vi "Stop Core.vi"(10 "final error code":i32, 11 "DataBase in":refnum<class "DataBase.lvclass">) -> (3 "DataBase out":refnum<class "DataBase.lvclass">)   [LabVIEW 2019, in "DataBase.lvlib" / "DataBase.lvclass"]
doc: "(<B>Filename</B>: Actor Framework.lvlib:Actor.lvclass:Stop Core.vi)\n\nDefines what the actor does before it stops. Use the <B>final error code</B> input to determine whether the actor shut down in response to an error.\n\nBy default, this method passes the Stop message along to all auto-stop nested actors. A descendant class may override this method to define additional behavior, such as shutting down any processes the actor initiated in its override of the Actor Core method."
uses:
  DataBase.lvclass
  DataBase.lvclass/DataBase.ctl
  79d7bb73-9b32-4418-8980-8c007c1ce44f.vi
  <vilib>/NI/Event Source Actor/Event Source/Event Source/Event Source.lvclass
  <vilib>/addons/database/NI_Database_API.lvlib
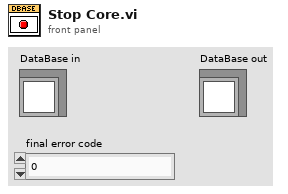
[diagram p1: front panel]
types:
  T1 = typedef "NI_Database_API.lvlib/Conn ObjectReference.ctl" = refnum<k1>
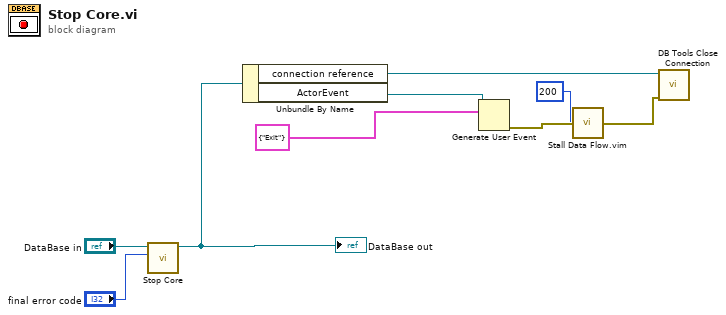
[diagram p0: block diagram]
diagram:
  n1 = call-parent "Stop Core.vi"("final error code"="final error code", "Event Source In"="DataBase in") -> ("Event Source Out"=w7:refnum<class "DataBase.lvclass">)  [unwired: 9 in]
  "DataBase out" <- w7
  n2 = Unbundle By Name(w7) -> ("connection reference"=w4:T1, "ActorEvent"=w6:refnum<user-event>)
  n3 = Generate User Event(user event=w6, event data cluster=cluster{"Message":string} {"Message"="Exit"} ("event data")) -> (error out=w3:errorcluster)  [unwired: 2 in, 1 out]
  n4 = call "Stall Data Flow.vim"("value in"=w3, "milliseconds to wait"=u32 200) -> ("value out"=w2:errorcluster)  [unwired: 1 out]
  n5 = call <vilib>:"DB Tools Close Connection.vi"("error in (no error)"=w2, "connection reference"=w4) -> ()  [unwired: 5 in, 1 out]
